vi "98-pubilc-html报表生成-精确时间及模糊时间命_带天数.vi"(10 "时间字符串输入":string) -> (0 "时分秒毫秒时间":string, 2 "天数":i32, 3 "带年日带毫秒时间":string, 5 "年月日":string)   [LabVIEW 2015]
panel:
  out "分钟":string
  out "长度 2":i32
  out "数字 3":i32
  out "数字 2":i32
  out "数字":i32
  out "长度":i32
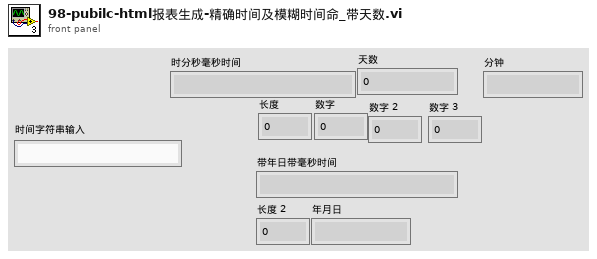
[diagram p1: front panel]
types:
  T1 = typedef "LVDateTimeRec.ctl" = cluster{"秒数的小数部分":dbl, "秒":i32, "分":i32, "时":i32, "日":i32, "月":i32, "年":i32, "天数（周）":i32, "天数（年）":i32, "DST":i32}
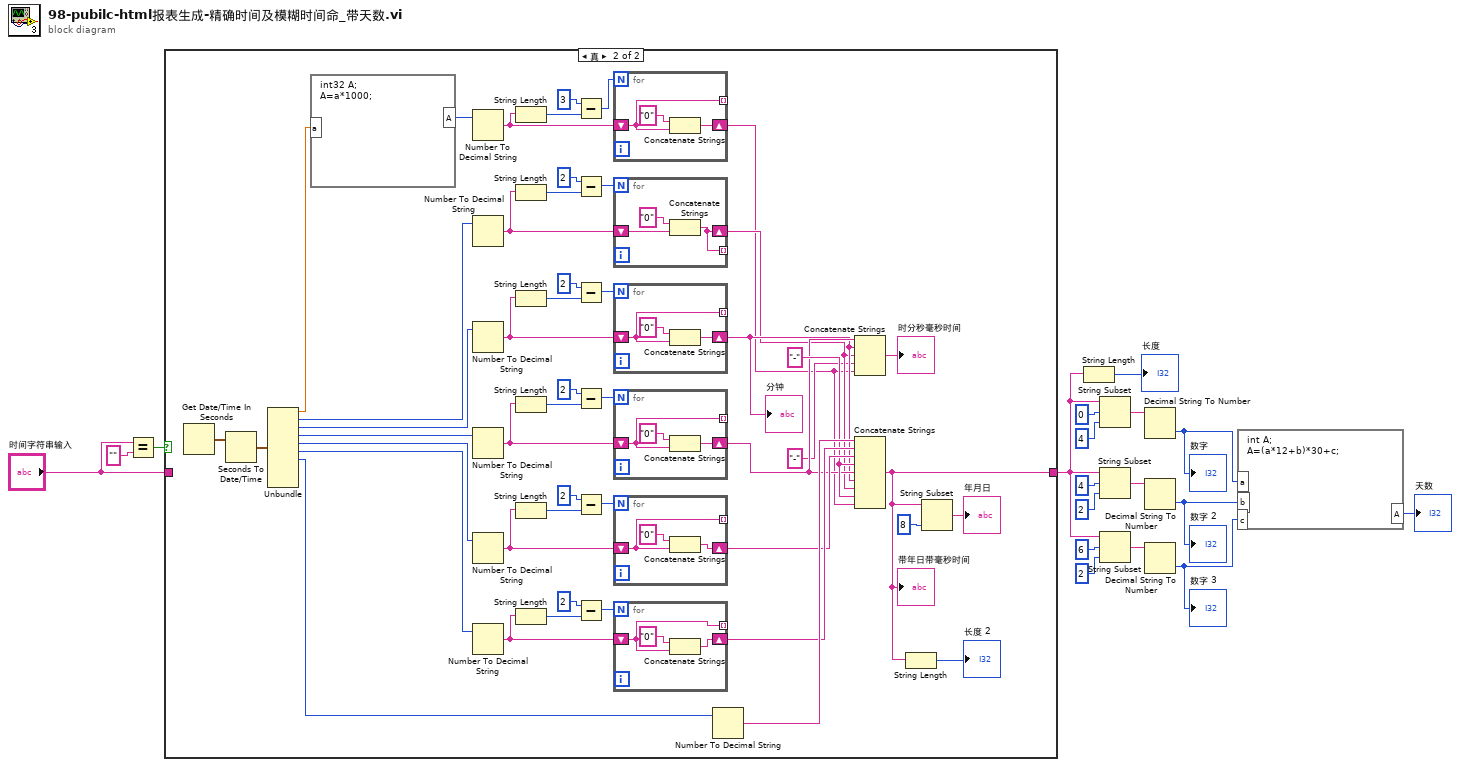
[diagram p0: block diagram]
diagram:
  n1 = Equal?(x="时间字符串输入", y="") -> (x = y?=w2:bool)
  n2 = case shown="真" w2 {
    tunnel: [w19 w22] -> w17
    tunnel: "时间字符串输入" -> [w19 _]
    frame False {
    }
    frame True {
      w30 = "-" ("字符串")
      n3 = Get Date/Time In Seconds() -> (seconds since 1Jan1904=w67:timestamp)
      n4 = Seconds To Date/Time(time stamp (now)=w67) -> (date time rec=w66:T1)  [unwired: 1 in]
      n5 = Unbundle(w66) -> ("秒数的小数部分"=w32:dbl, "秒"=w37:i32, "分"=w42:i32, "时"=w47:i32, "日"=w53:i32, "月"=w63:i32, "年"=w65:i32)  [unwired: 3 out]
      n6 = formula code="int32 A;\nA=a*1000;"("a"=w32) -> ("A"=w31:i32)
      n7 = Number To Decimal String(number=w31) -> (decimal integer string=w33:string)  [unwired: 1 in]
      n8 = Number To Decimal String(number=w37) -> (decimal integer string=w38:string)  [unwired: 1 in]
      n9 = Number To Decimal String(number=w42) -> (decimal integer string=w43:string)  [unwired: 1 in]
      n10 = Number To Decimal String(number=w47) -> (decimal integer string=w48:string)  [unwired: 1 in]
      n11 = Number To Decimal String(number=w53) -> (decimal integer string=w54:string)  [unwired: 1 in]
      n12 = Number To Decimal String(number=w63) -> (decimal integer string=w60:string)  [unwired: 1 in]
      n13 = String Length(string=w33) -> (length=w35:i32)
      n14 = String Length(string=w38) -> (length=w40:i32)
      n15 = String Length(string=w43) -> (length=w45:i32)
      n16 = String Length(string=w48) -> (length=w50:i32)
      n17 = String Length(string=w54) -> (length=w56:i32)
      n18 = String Length(string=w60) -> (length=w62:i32)
      n19 = Subtract(x=3, y=w35) -> (x-y=w34:i32)
      n20 = Subtract(x=2, y=w40) -> (x-y=w39:i32)
      n21 = Subtract(x=2, y=w45) -> (x-y=w44:i32)
      n22 = Subtract(x=2, y=w50) -> (x-y=w49:i32)
      n23 = Subtract(x=2, y=w56) -> (x-y=w55:i32)
      n24 = Subtract(x=2, y=w62) -> (x-y=w61:i32)
      n25 = for {
        N: w34 -> [_]
        shift-right: [w69] -> w25
        shift-left: w33 -> [w68]
        tunnel: [w68] -> _ mode=indexing
        n26 = Concatenate Strings("0" ("字符串"), w68) -> (w69:string)
      }
      n27 = for {
        N: w39 -> [_]
        shift-right: [w71] -> w27
        shift-left: w38 -> [w72]
        tunnel: [w71] -> _ mode=indexing
        n28 = Concatenate Strings("0" ("字符串"), w72) -> (w71:string)
      }
      n29 = for {
        N: w44 -> [_]
        shift-right: [w75] -> w28
        shift-left: w43 -> [w74]
        tunnel: [w74] -> _ mode=indexing
        n30 = Concatenate Strings("0" ("字符串"), w74) -> (w75:string)
      }
      "分钟" <- w28
      n31 = for {
        N: w49 -> [_]
        shift-right: [w78] -> w29
        shift-left: w48 -> [w77]
        tunnel: [w77] -> _ mode=indexing
        n32 = Concatenate Strings("0" ("字符串"), w77) -> (w78:string)
      }
      n33 = for {
        N: w55 -> [_]
        shift-right: [w81] -> w52
        shift-left: w54 -> [w80]
        tunnel: [w80] -> _ mode=indexing
        n34 = Concatenate Strings("0" ("字符串"), w80) -> (w81:string)
      }
      n35 = for {
        N: w61 -> [_]
        shift-right: [w84] -> w58
        shift-left: w60 -> [w83]
        tunnel: [w83] -> _ mode=indexing
        n36 = Concatenate Strings("0" ("字符串"), w83) -> (w84:string)
      }
      n37 = Number To Decimal String(number=w65) -> (decimal integer string=w59:string)  [unwired: 1 in]
      n38 = Concatenate Strings(w29, w28, w27, "-" ("字符串"), w25) -> (→"时分秒毫秒时间":string)
      n39 = Concatenate Strings(w59, w58, w52, w30, w29, w28, w27, w30, w25) -> (w22:string)
      "带年日带毫秒时间" <- w22
      n40 = String Length(string=w22) -> (length=→"长度 2":i32)
      n41 = String Subset(string=w22, length (rest)=8 ("长度（剩余）")) -> (substring=→"年月日":string)  [unwired: 1 in]
    }
  }
  n42 = String Length(string=w17) -> (length=→"长度":i32)
  n43 = String Subset(string=w17, offset (0)=0 ("偏移量(0)"), length (rest)=4 ("长度（剩余）")) -> (substring=w10:string)
  n44 = String Subset(string=w17, offset (0)=4 ("偏移量(0)"), length (rest)=2 ("长度（剩余）")) -> (substring=w8:string)
  n45 = String Subset(string=w17, offset (0)=6 ("偏移量(0)"), length (rest)=2 ("长度（剩余）")) -> (substring=w6:string)
  n46 = Decimal String To Number(string=w10) -> (number=w9:i32)  [unwired: 2 in, 1 out]
  "数字" <- w9
  n47 = Decimal String To Number(string=w8) -> (number=w7:i32)  [unwired: 2 in, 1 out]
  "数字 2" <- w7
  n48 = Decimal String To Number(string=w6) -> (number=w5:i32)  [unwired: 2 in, 1 out]
  "数字 3" <- w5
  n49 = formula code="int A;\nA=(a*12+b)*30+c;"("a"=w9, "b"=w7, "c"=w5) -> ("A"=→"天数":i32)
